vi "Untitled 3.vi"() -> ()   [LabVIEW 2019]
panel:
  out "*(type *) &x 4":u32
  out "*(type *) &x 3":u32
  out "*(type *) &x":u32
  out "*(type *) &x 2":string
  out "substring":string
  out "name":string
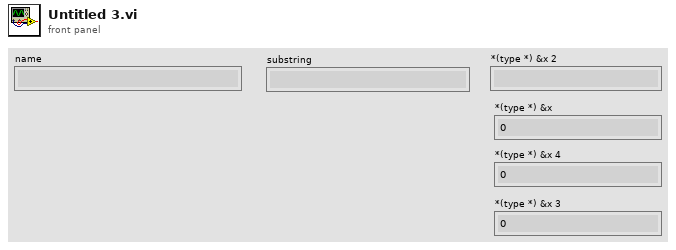
[diagram p1: front panel]
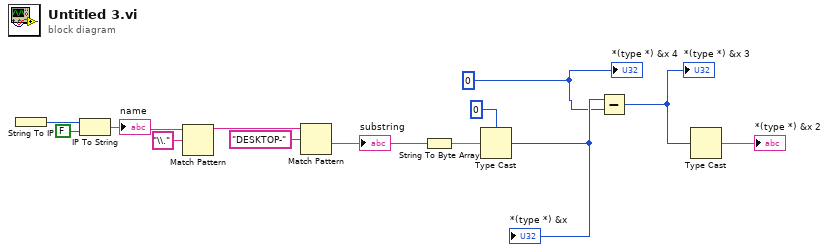
[diagram p0: block diagram]
diagram:
  w1 = u32 0 ("ChassisSerialNumber")
  n1 = String To IP() -> (0:w13:u32)  [unwired: 1 in]
  n2 = IP To String(1:FALSE ("dot notation? (F)"), 2:w13) -> (0:w12:string)
  "name" <- w12
  n3 = Match Pattern(string=w12, regular expression="\\.") -> (before substring=w5:string)  [unwired: 1 in, 3 out]
  n4 = Match Pattern(string=w5, regular expression="DESKTOP-") -> (after substring=w4:string)  [unwired: 1 in, 3 out]
  "substring" <- w4
  n5 = String To Byte Array(string=w4) -> (unsigned byte array=w9:u8[])
  n6 = Type Cast(type=u32 0, x=w9) -> (*(type *) &x=w3:u32)
  "*(type *) &x" <- w3
  n7 = Subtract(x=w3, y=w1) -> (x-y=w2:u32)
  "*(type *) &x 3" <- w2
  n8 = Type Cast(x=w2) -> (*(type *) &x=→"*(type *) &x 2":string)  [unwired: 1 in]
  "*(type *) &x 4" <- w1
